vi "readFromXML.vi"(8 "error in (no error)":errorcluster, 10 "XML in":string, 11 "PointNew in":refnum<class "PointNew.lvclass">) -> (0 "error out":errorcluster, 3 "PointNew out":refnum<class "PointNew.lvclass">)   [LabVIEW 2022 SP3, in "TCSDataDefinitions.lvlib" / "TCSCommand.lvlib" / "PointingFileCommands.lvlib" / "PointNew.lvclass"]
uses:
  PointNew.lvclass
  PointingFileCommands/PointingFileCommands.lvclass
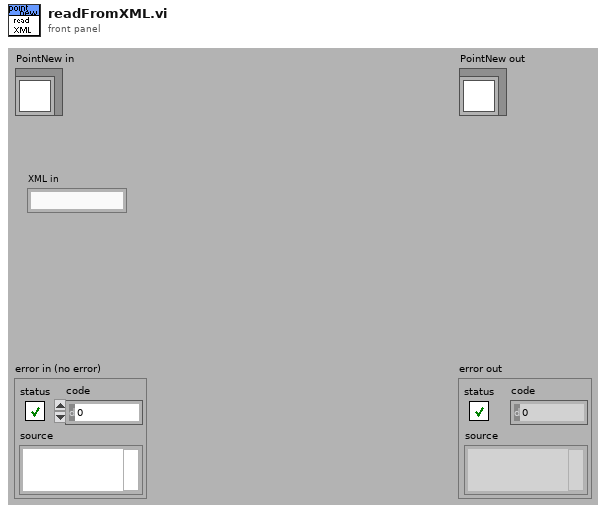
[diagram p1: front panel]
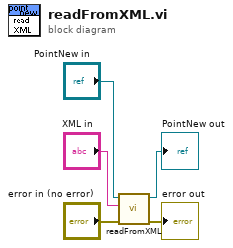
[diagram p0: block diagram]
diagram:
  n1 = call-parent "readFromXML.vi"("error in (no error)"="error in (no error)", "XML in"="XML in", "PointingFileCommands in"="PointNew in") -> ("error out"=→"error out":errorcluster, "PointingFileCommands out"=→"PointNew out":refnum<class "PointNew.lvclass">)  [unwired: 7 out]
